vi "WriteValueToQueueDisplay.vi"(0 "XuLyStringUART in":refnum<class "XuLyStringUART.lvclass">, 3 "error in (no error)":errorcluster, 4 "Writepara":enum16{"Config", "Pos"}(ring)) -> (7 "XuLyStringUART out":refnum<class "XuLyStringUART.lvclass">, 10 "error out":errorcluster)   [LabVIEW 2014, in "LibraryGcode.lvlib" / "XuLyStringUART.lvclass"]
uses:
  XuLyStringUART.lvclass
  control/stateCmdUpdatePara.ctl
  XuLyStringUART.lvclass/XuLyStringUART.ctl
  LibraryGcode.lvlib
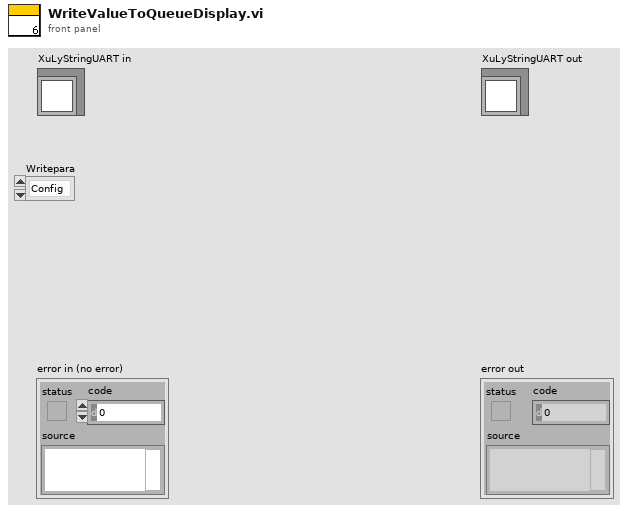
[diagram p1: front panel]
types:
  T1 = typedef "LibraryGcode.lvlib/stateCmdUpdatePara.ctl" = enum16{"updatePos", "UpdateConfigAccel", "UpdateConfigFeed", "UpdateConfigUnit", "UpdateConfigStartAccel", "NoUpdate"}
  T2 = cluster{"Command":T1, "POS":cluster{"X":dbl, "Y":dbl, "Z":dbl}, "DEGREES":cluster{"X":dbl, "Y":dbl}}
  T3 = typedef "LibraryGcode.lvlib/XuLyStringUART.lvclass/ListMcodeConfig.ctl" = enum16{"M203", "M201", "M92", "M3001", "M204"}
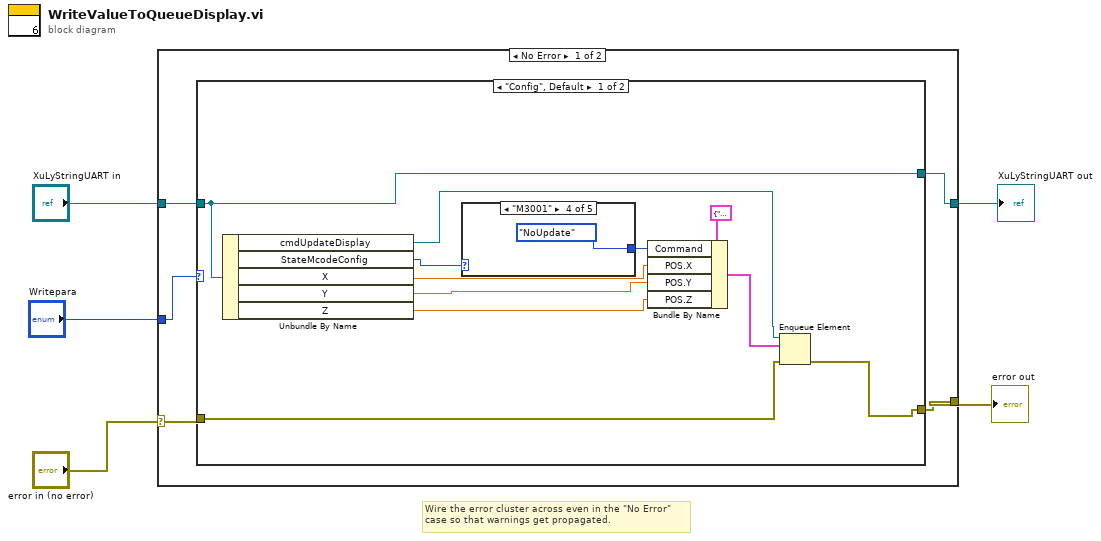
[diagram p0: block diagram]
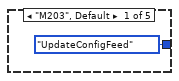
[diagram p2: hidden frame]
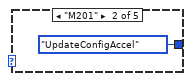
[diagram p3: hidden frame]
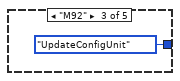
[diagram p4: hidden frame]
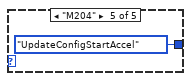
[diagram p5: hidden frame]
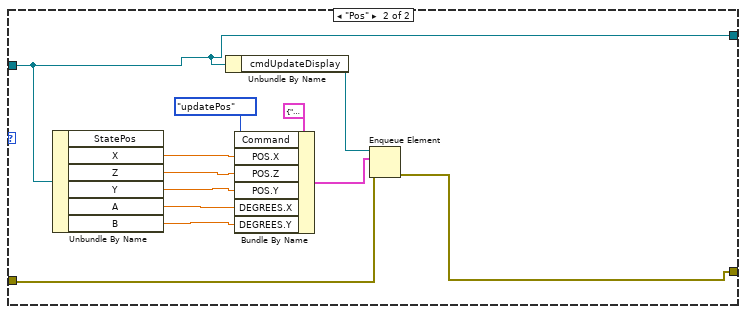
[diagram p6: hidden frame]
diagram:
  # "Wire the error cluster across even in the \"No Error\"\ncase so that warnings get propagated."
  n1 = case shown="No Error" "error in (no error)" {
    selector: "error in (no error)" -> [w10 w40]
    tunnel: [w8 w40] -> w4
    tunnel: [w6 w39] -> w3
    tunnel: "XuLyStringUART in" -> [w9 w39]
    tunnel: "Writepara" -> [w7 _]
    frame No Error {
      n2 = case shown="\"Config\", Default" w7 {
        tunnel: w10 -> [w16 w38]
        tunnel: [w15 w27] -> w8
        tunnel: w9 -> [w11 w28]
        tunnel: [w11 w28] -> w6
        frame "Config", Default {
          n3 = Unbundle By Name(w11) -> ("cmdUpdateDisplay"=w17:refnum<queue>, "StateMcodeConfig"=w21:T3, "X"=w14:dbl, "Y"=w13:dbl, "Z"=w12:dbl)
          n4 = case shown="\"M3001\"" w21 {
            tunnel: [stateCmdUpdatePara."UpdateConfigFeed" ("Command") stateCmdUpdatePara."UpdateConfigAccel" ("Command") stateCmdUpdatePara."UpdateConfigUnit" ("Command") stateCmdUpdatePara."NoUpdate" ("Command") stateCmdUpdatePara."UpdateConfigStartAccel" ("Command")] -> w18
            frame "M203", Default {
            }
            frame "M201" {
            }
            frame "M92" {
            }
            frame "M3001" {
            }
            frame "M204" {
            }
          }
          n5 = Bundle By Name(cluster=T2 {"Command"=enum."updatePos", "POS"={"X"=0.0, "Y"=0.0, "Z"=0.0}, "DEGREES"={"X"=0.0, "Y"=0.0}} ("element"), "Command"=w18, "POS.X"=w14, "POS.Y"=w13, "POS.Z"=w12) -> (w19:T2)
          n6 = Enqueue Element(queue=w17, element=w19, error in (no error)=w16) -> (error out=w15:errorcluster)  [unwired: 1 in, 2 out]
        }
        frame "Pos" {
          n7 = Unbundle By Name(w28) -> ("X"=w33:dbl, "Z"=w32:dbl, "Y"=w31:dbl, "A"=w30:dbl, "B"=w29:dbl)  [unwired: 1 out]
          n8 = Unbundle By Name(w28) -> ("cmdUpdateDisplay"=w35:refnum<queue>)
          n9 = Bundle By Name(cluster=T2 {"Command"=enum."updatePos", "POS"={"X"=0.0, "Y"=0.0, "Z"=0.0}, "DEGREES"={"X"=0.0, "Y"=0.0}} ("element"), "Command"=stateCmdUpdatePara."updatePos", "POS.X"=w33, "POS.Z"=w32, "POS.Y"=w31, "DEGREES.X"=w30, "DEGREES.Y"=w29) -> (w36:T2)
          n10 = Enqueue Element(queue=w35, element=w36, error in (no error)=w38) -> (error out=w27:errorcluster)  [unwired: 1 in, 2 out]
        }
      }
    }
    frame Error {
    }
  }
  "error out" <- w4
  "XuLyStringUART out" <- w3
